vi "Memory Game Part 4.vi"() -> ()   [LabVIEW 2019]
uses:
  <vilib>/numeric/Random Number (Range) U64.vi
panel:
  in  "Keys":T1
  out "Number of the correct dials":i32
  out "Display":u32(colorbox) caption="Sequence to memorise"
  # "Memory Mobile Game"
  # "Dial the number shown in the display"
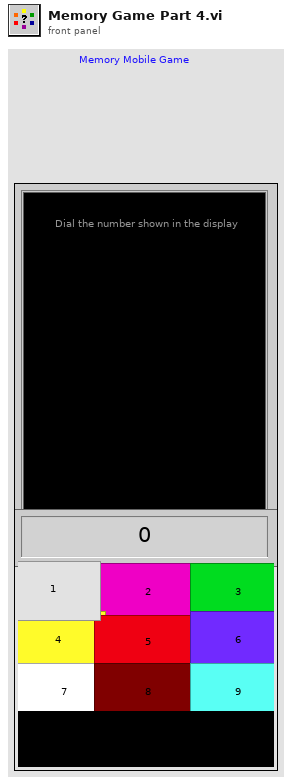
[diagram p1: front panel]
types:
  T1 = cluster{"0":bool, "1":bool, "2":bool, "3":bool, "4":bool, "5":bool, "6":bool, "7":bool, "8":bool, "9":bool}
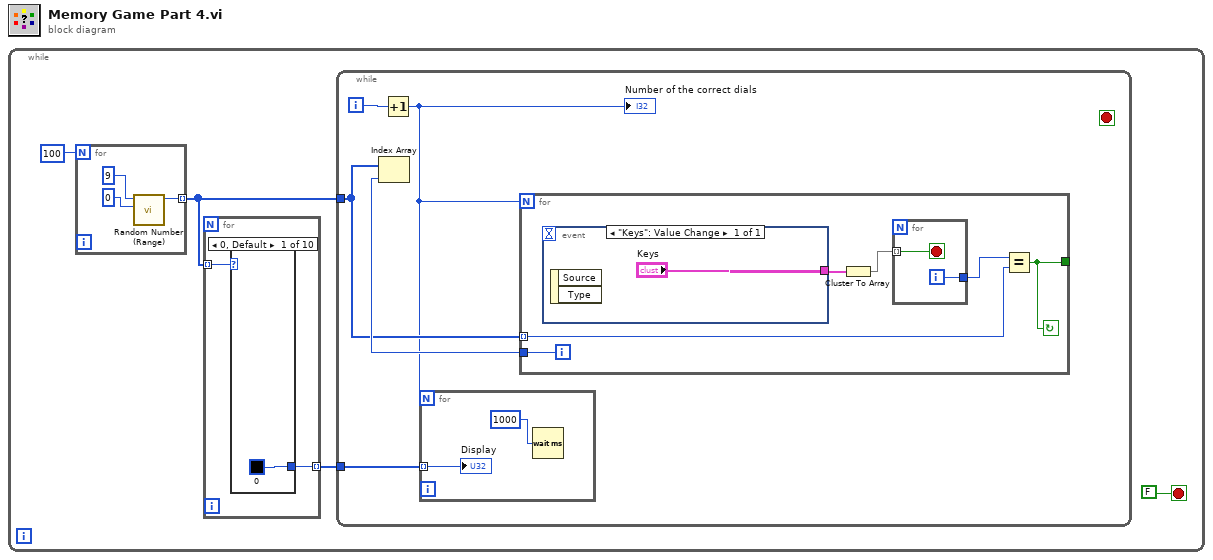
[diagram p0: block diagram]
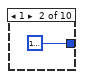
[diagram p2: hidden frame]
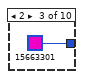
[diagram p3: hidden frame]
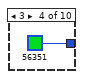
[diagram p4: hidden frame]
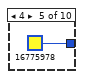
[diagram p5: hidden frame]
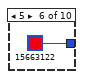
[diagram p6: hidden frame]
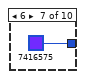
[diagram p7: hidden frame]
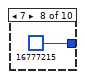
[diagram p8: hidden frame]
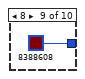
[diagram p9: hidden frame]
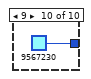
[diagram p10: hidden frame]
diagram:
  n1 = while {
    stop <- FALSE stop-if-true
    # "Main loop, run  once per game"
    n2 = for {
      N: 100 -> [_]
      tunnel: [w17] -> w2 mode=indexing
      # "generate randome sequence of\ncolor indices (0 .. 9)"
      n3 = call-poly <vilib>:"Random Number (Range).vi"("lower bound (0)"=u64 0, "upper bound (100)"=u64 9) -> ("number"=w17:u64)  [unwired: 9 in]
    }
    n4 = for {
      tunnel: w2 -> [w6] mode=indexing
      tunnel: [w5] -> w1 mode=indexing
      # "generate sequence of colors"
      n5 = case shown="0, Default" w6 {
        tunnel: [u32 0 ("Color Box") u32 16777224 ("Color Box") u32 15663301 ("Color Box") u32 56351 ("Color Box") u32 16775978 ("Color Box") u32 15663122 ("Color Box") u32 7416575 ("Color Box") u32 16777215 ("Color Box") u32 8388608 ("Color Box") u32 9567230 ("Color Box")] -> w5
        frame 0, Default {
        }
        frame 1 {
        }
        frame 2 {
        }
        frame 3 {
        }
        frame 4 {
        }
        frame 5 {
        }
        frame 6 {
        }
        frame 7 {
        }
        frame 8 {
        }
        frame 9 {
        }
      }
    }
    n6 = while {
      tunnel: w2 -> [w22]
      tunnel: w1 -> [w21]
      i -> [w23]
      stop <- _ stop-if-true
      # "Check input of sequnece"
      n7 = Increment(x=w23) -> (x+1=w20:i32)
      "Number of the correct dials" <- w20
      n8 = for {
        N: w20 -> [_]
        tunnel: w21 -> [w25] mode=indexing
        # "play sequence"
        n9 = Wait (ms)(milliseconds to wait=u32 1000 ("Zu wartende ms")) -> ()  [unwired: 1 out]
        "Display" <- w25
      }
      n10 = for {
        N: w20 -> [_]
        tunnel: w22 -> [w29] mode=indexing
        tunnel: [w28] -> _
        tunnel: [w27] -> w24
        i -> [w27]
        stop <- w28 continue-if-true
        # "Get and check user input"
        n11 = event shown="[0] \"Keys\": Value Change" {
          selector: _ -> [_]
          dyn-events: _ -> [_]
          timeout: _ -> [_]
          tunnel: ["Keys"] -> w32
          event "Keys": Value Change {
            n12 = event-data() -> ()  [unwired: 1 in, 2 out]
          }
        }
        n13 = Cluster To Array(cluster=w32) -> (array=w31:bool[])
        n14 = for {
          tunnel: w31 -> [w34] mode=indexing
          tunnel: [w33] -> w30
          i -> [w33]
          stop <- w34 stop-if-true
        }
        n15 = Equal?(x=w30, y=w29) -> (x = y?=w28:bool)
      }
      n16 = Index Array "Index Array"(array=w22, index=w24) -> ()  [unwired: 1 out]
    }
  }
